vi "Configure Source Advanced Sequence Mode.vi"(0 "Instrument handle IN":refnum<k15>[](array[refnum]), 1 "Measurement Configuration":T2={"Quick Power Down"=FALSE, "Pin Name"=[], "Source Mode"=[], "Start Value"=[], "Target Value"=[], "Compliance Limit"=[], "Sense Mode"=[], "Default Ramp Rate"=[], "Ramp Rate"=[], "Start Delay"=[], "Relative To"=[], "Transient Response"=[], "Data Capture"=FALSE, "Power line frequency"=1} {"Power line frequency" items=["50 Hz", "60 Hz"]; "Start Value" format="%#_6p"; "Transient Response" items=["Slow", "Normal", "Fast"]; "Sense Mode" items=["Local Sense", "Remote Sense"]; "Relative To" items=["Power sequence start", "Previous source start", "Previous source end"]; "Target Value" format="%#_6p"; "Source Mode" items=["DC Voltage", "DC Current"]; "Start Delay" format="%#_6p"; "Compliance Limit" format="%#_6p"; "Ramp Rate" format="%#_6p"}, 2 "PowerUP?":bool, 5 "Channel Number":string[](array[string]), 7 "Ramp Configurations":T1, 11 "error in (no error)":errorcluster) -> (4 "Instrument Handle OUT":refnum<k15>[](array[refnum]), 6 "Advance Seq Created?":bool[](array[boolean]), 15 "error out":errorcluster)   [LabVIEW 2024, in "devicePowerSequencerCoreLogic.lvlib"]
uses:
  devicePowerSequencerCoreLogic.lvlib
  Measurement Configuration.ctl
  controls/Source Mode.ctl
  controls/Sense Mode.ctl
  controls/Relative To.ctl
  controls/Transient Response.ctl
  controls/Power line frequency.ctl
  controls/Ramp Configurations.ctl
  <instrlib>/niDCPower/nidcpower.llb/niDCPower Sequence Attribute Type.ctl
  <vilib>/Analysis/1siggen.llb/Ramp Pattern by Samples.vi
  <instrlib>/niDCPower/nidcpower.llb/niDCPower Create Advanced Sequence Commit Step With Channels.vi
  <instrlib>/niDCPower/nidcpower.llb/niDCPower Create Advanced Sequence Step With Channels.vi
  <vilib>/Analysis/NI_AALBase.lvlib
  Device Power Sequencer.lvlib
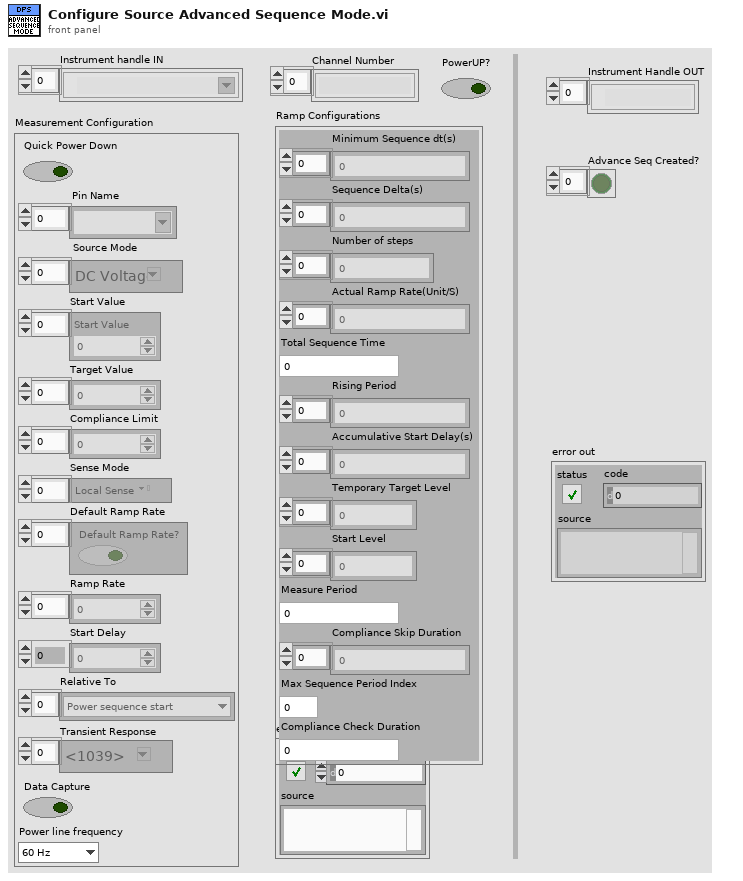
[diagram p1: front panel]
types:
  T1 = typedef "devicePowerSequencerCoreLogic.lvlib/Ramp Configurations.ctl" = cluster{"Minimum Sequence dt(s)":dbl[], "Sequence Delta(s)":dbl[], "Number of steps":i32[], "Actual Ramp Rate(Unit/S)":dbl[], "Total Sequence Time":dbl, "Rising Period":dbl[], "Accumulative Start Delay(s)":dbl[], "Temporary Target Level":dbl[], "Start Level":dbl[], "Measure Period":dbl, "Compliance Skip Duration":dbl[], "Max Sequence Period Index":i32, "Compliance Check Duration":dbl}
  T2 = typedef "Device Power Sequencer.lvlib/Measurement Configuration.ctl" = cluster{"Quick Power Down":bool, "Pin Name":string[], "Source Mode":T3[], "Start Value":dbl[], "Target Value":dbl[], "Compliance Limit":dbl[], "Sense Mode":T4[], "Default Ramp Rate":bool[], "Ramp Rate":dbl[], "Start Delay":dbl[], "Relative To":T5[], "Transient Response":T6[], "Data Capture":bool, "Power line frequency":T7}
  T3 = typedef "Device Power Sequencer.lvlib/Source Mode.ctl" = i32
  T4 = typedef "Device Power Sequencer.lvlib/Sense Mode.ctl" = i32
  T5 = typedef "Device Power Sequencer.lvlib/Relative To.ctl" = u32
  T6 = typedef "Device Power Sequencer.lvlib/Transient Response.ctl" = i32
  T7 = typedef "Device Power Sequencer.lvlib/Power line frequency.ctl" = u32
  T8 = typedef "niDCPower Sequence Attribute Type.ctl" = i32
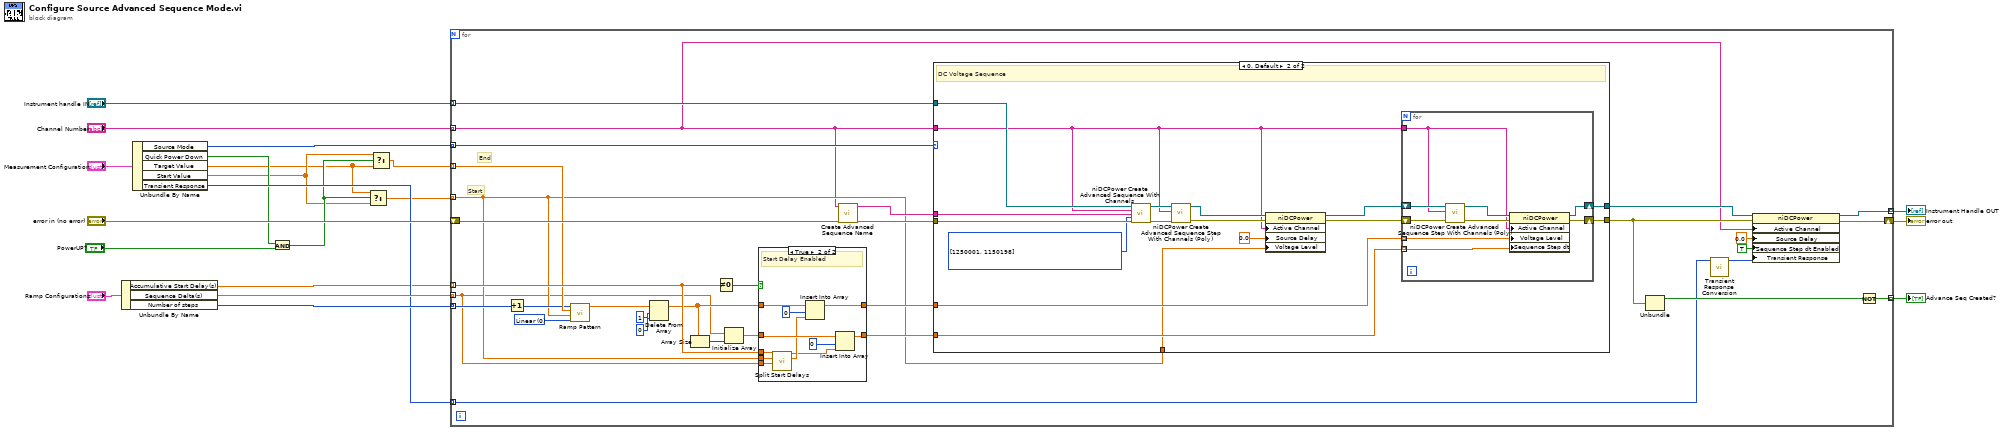
[diagram p0: block diagram]
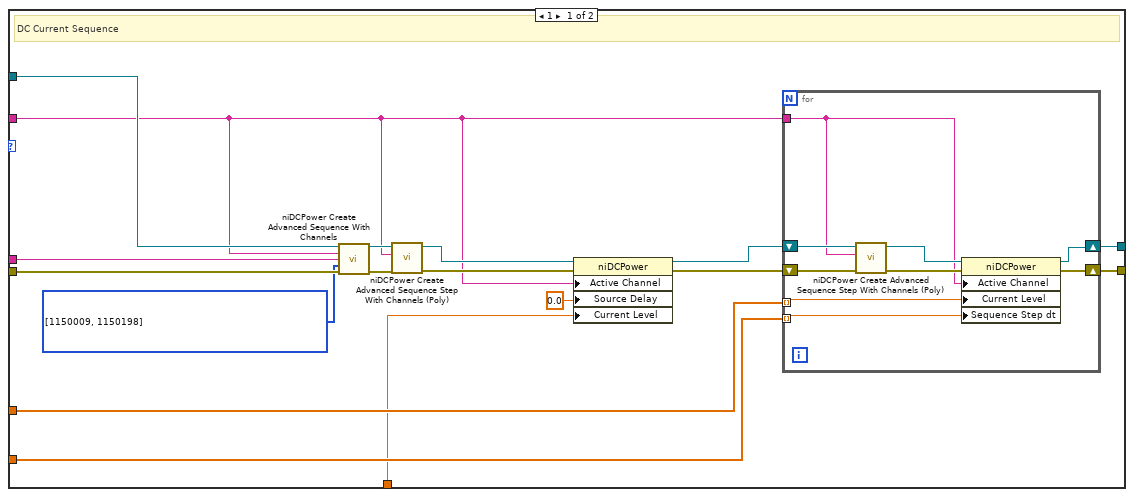
[diagram p3: hidden frame]
diagram:
  n1 = Unbundle By Name("Ramp Configurations") -> ("Accumulative Start Delay(s)"=w8:dbl[], "Sequence Delta(s)"=w15:dbl[], "Number of steps"=w17:i32[])
  n2 = Unbundle By Name("Measurement Configuration") -> ("Source Mode"=w16:T3[], "Quick Power Down"=w4:bool, "Target Value"=w1:dbl[], "Start Value"=w2:dbl[], "Transient Response"=w9:T6[])
  n3 = And(x=w4, y="PowerUP?") -> (x .and. y?=w5:bool)
  n4 = Select(t=w1, s=w5, f=w2) -> (s? t:f=w6:dbl[])
  n5 = Select(t=w2, s=w5, f=w1) -> (s? t:f=w7:dbl[])
  n6 = for {
    tunnel: "Instrument handle IN" -> [w51] mode=indexing
    tunnel: w17 -> [w52] mode=indexing
    tunnel: w7 -> [w37] mode=indexing
    tunnel: w8 -> [w38] mode=indexing
    tunnel: w16 -> [w48] mode=indexing
    tunnel: w15 -> [w22] mode=indexing
    tunnel: "Channel Number" -> [w21] mode=indexing
    shift-right: [w42] -> w12
    shift-left: "error in (no error)" -> [w44]
    tunnel: [w43] -> w11 mode=indexing
    tunnel: [w41] -> w10 mode=indexing
    tunnel: w9 -> [w27] mode=indexing
    tunnel: w6 -> [w23] mode=indexing
    w34 = u16 0 items=["Linear", "Logarithmic"] ("type")
    # "End"
    # "Start"
    n7 = Increment(x=w52) -> (x+1=w35:i32)
    n8 = call-poly <vilib>:"Ramp Pattern.vi"("type"=w34, "start"=w23, "end"=w37, "samples"=w35) -> ("Ramp Pattern"=w28:dbl[])  [unwired: 6 in, 1 out]
    n9 = Delete From Array(array=w28, length=1, index=0) -> (array with subset deleted=w31:dbl[])  [unwired: 1 out]
    n10 = Array Size(array=w31) -> (size(s)=w30:i32)
    n11 = Not Equal To 0?(x=w38) -> (x != 0?=w36:bool)
    n12 = Initialize Array(w22, w30) -> (w29:dbl[])
    n13 = case shown="True" w36 {
      tunnel: w31 -> [w54 w64]
      tunnel: [w54 w63] -> w25
      tunnel: w29 -> [w53 w60]
      tunnel: [w53 w61] -> w24
      tunnel: w38 -> [_ w59]
      tunnel: w23 -> [_ w58]
      tunnel: w22 -> [_ w55]
      frame False {
      }
      frame True {
        # "Start Delay Enabled"
        n14 = call "Split Start Delays.vi"("Start Delay"=w59, "Value"=w58, "Sequence Delta (s)"=w55) -> ("Start Delay"=w56:dbl[], "Value"=w57:dbl[])  [unwired: 11 in]
        n15 = Insert Into Array(array=w64, index=0, new element=w57) -> (w63:dbl[])
        n16 = Insert Into Array(array=w60, index=0, new element=w56) -> (w61:dbl[])
      }
    }
    n17 = call "Create Advanced Sequence Name.vi"("Channel Name"=w21, "error in (no error)"=w44) -> ("String"=w49:string, "error out"=w50:errorcluster)  [unwired: 12 in]
    n18 = case shown="0, Default" w48 {
      tunnel: w51 -> [w82 w108]
      tunnel: w50 -> [w81 w107]
      tunnel: w49 -> [w80 w106]
      tunnel: [w74 w97] -> w47
      tunnel: w25 -> [w73 w96]
      tunnel: w24 -> [w72 w95]
      tunnel: w21 -> [w66 w92]
      tunnel: [w71 w94] -> w39
      tunnel: w23 -> [w67 w93]
      frame 1 {
        w77 = T8[] [1150009, 1150198] items=["Source -> Output Function"=1150008, "Source -> Output Enabled"=1250006, "Source -> Output Resistance"=1150061, "Source -> Transient Response"=1150062, "Source -> Custom Transient Response -> Voltage Gain Bandwidth"=1150067, "Source -> Custom Transient Response -> Voltage Compensation Frequency"=1150068, "Source -> Custom Transient Response -> Voltage Pole-Zero Ratio"=1150069, "Source -> Custom Transient Response -> Current Gain Bandwidth"=1150070, "Source -> Custom Transient Response -> Current Compensation Frequency"=1150071, "Source -> Custom Transient Response -> Current Pole-Zero Ratio"=1150072, "Source -> DC Voltage -> Voltage Level"=1250001, "Source -> DC Voltage -> Voltage Level Range"=1150005, "Source -> DC Voltage -> Current Limit"=1250005, "Source -> DC Voltage -> Current Limit High"=1150187, "Source -> DC Voltage -> Current Limit Low"=1150188, "Source -> DC Voltage -> Current Limit Range"=1150004, "Source -> DC Current -> Current Level"=1150009, "Source -> DC Current -> Current Level Range"=1150011, "Source -> DC Current -> Voltage Limit"=1150010, "Source -> DC Current -> Voltage Limit High"=1150185, "Source -> DC Current -> Voltage Limit Low"=1150186, "Source -> DC Current -> Voltage Limit Range"=1150012, "Source -> Pulse Voltage -> Pulse Voltage Level"=1150080, "Source -> Pulse Voltage -> Pulse Bias Voltage Level"=1150082, "Source -> Pulse Voltage -> Pulse Voltage Level Range"=1150084, "Source -> Pulse Voltage -> Pulse Current Limit"=1150081, "Source -> Pulse Voltage -> Pulse Current Limit High"=1150193, "Source -> Pulse Voltage -> Pulse Current Limit Low"=1150194, "Source -> Pulse Voltage -> Pulse Bias Current Limit"=1150083, "Source -> Pulse Voltage -> Pulse Bias Current Limit High"=1150195, "Source -> Pulse Voltage -> Pulse Bias Current Limit Low"=1150196, "Source -> Pulse Voltage -> Pulse Current Limit Range"=1150085, "Source -> Pulse Current -> Pulse Current Level"=1150086, "Source -> Pulse Current -> Pulse Bias Current Level"=1150088, "Source -> Pulse Current -> Pulse Current Level Range"=1150090, "Source -> Pulse Current -> Pulse Voltage Limit"=1150087, "Source -> Pulse Current -> Pulse Voltage Limit High"=1150189, "Source -> Pulse Current -> Pulse Voltage Limit Low"=1150190, "Source -> Pulse Current -> Pulse Bias Voltage Limit"=1150089, "Source -> Pulse Current -> Pulse Bias Voltage Limit High"=1150191, "Source -> Pulse Current -> Pulse Bias Voltage Limit Low"=1150192, "Source -> Pulse Current -> Pulse Voltage Limit Range"=1150091, "Source -> Advanced -> Source Delay"=1150051, "Source -> Advanced -> Pulse Bias Delay"=1150092, "Source -> Advanced -> Pulse On Time"=1150093, "Source -> Advanced -> Pulse Off Time"=1150094, "Source -> Advanced -> OVP Enabled"=1250002, "Source -> Advanced -> OVP Limit"=1250003, "Source -> Advanced -> Compliance Limit Symmetry"=1150184, "Source -> Advanced -> Sequence Step Delta Time"=1150198, "Measurement -> Sense"=1150013, "Measurement -> Aperture Time"=1150058, "Measurement -> Measure Record Length"=1150063, "Measurement -> Advanced -> DC Noise Rejection"=1150066, "Measurement -> Autorange"=1150244, "Measurement -> Advanced -> Autorange Behavior"=1150245, "Measurement -> Advanced -> Autorange Aperture Time Mode"=1150246, "Measurement -> Advanced -> Autorange Minimum Aperture Time"=1150247, "Measurement -> Advanced -> Autorange Minimum Aperture Time Units"=1150248, "Measurement -> Advanced -> Autorange Minimum Current Range"=1150255, "Measurement -> Advanced -> Autorange Minimum Voltage Range"=1150256, "Measurement -> Advanced -> Autorange Threshold Mode"=1150257, "Measurement -> Advanced -> Autorange Maximum Delay After Range Change"=1150322, "LCR -> Instrument Mode"=1150208, "LCR -> Source Delay Mode"=1150315, "LCR -> Measurement Time"=1150218, "LCR -> Custom Measurement Time"=1150258, "LCR -> AC Stimulus -> Function"=1150209, "LCR -> AC Stimulus -> Frequency"=1150210, "LCR -> AC Stimulus -> Voltage Amplitude"=1150211, "LCR -> AC Stimulus -> Current Amplitude"=1150212, "LCR -> AC Stimulus -> Advanced -> Voltage Range"=1150265, "LCR -> AC Stimulus -> Advanced -> Current Range"=1150267, "LCR -> DC Bias -> Source"=1150213, "LCR -> DC Bias -> Voltage Level"=1150214, "LCR -> DC Bias -> Current Level"=1150215, "LCR -> DC Bias -> Advanced -> Voltage Range"=1150266, "LCR -> DC Bias -> Advanced -> Current Range"=1150274, "LCR -> Compensation -> Open -> Enabled"=1150220, "LCR -> Compensation -> Open -> Conductance"=1150261, "LCR -> Compensation -> Open -> Susceptance"=1150262, "LCR -> Compensation -> Short -> Enabled"=1150221, "LCR -> Compensation -> Short -> Resistance"=1150263, "LCR -> Compensation -> Short -> Reactance"=1150264, "LCR -> Compensation -> Load -> Enabled"=1150222, "LCR -> Compensation -> Load -> Measured Resistance"=1150268, "LCR -> Compensation -> Load -> Measured Reactance"=1150269, "LCR -> Compensation -> Load -> Actual Resistance"=1150270, "LCR -> Compensation -> Load -> Actual Reactance"=1150271, "LCR -> Impedance Range -> Impedance Range"=1150217, "LCR -> Impedance Range -> Impedance Autorange"=1150216, "LCR -> Impedance Range -> Advanced -> Impedance Range Source"=1150321, "LCR -> Impedance Range -> Advanced -> Load Resistance"=1150318, "LCR -> Impedance Range -> Advanced -> Load Inductance"=1150319, "LCR -> Impedance Range -> Advanced -> Load Capacitance"=1150320] ("advanced sequence properties")
        # "DC Current Sequence"
        n19 = call <instrlib>:"niDCPower Create Advanced Sequence With Channels.vi"("instrument handle"=w82, "channel name"=w66, "sequence name"=w80, "advanced sequence properties"=w77, "error in (no error)"=w81) -> ("instrument handle out"=w78:refnum<k15>, "error out"=w79:errorcluster)  [unwired: 9 in]
        n20 = call-poly <instrlib>:"niDCPower Create Advanced Sequence Step With Channels (Poly).vi"("error in (no error)"=w79, "channel name"=w66, "instrument handle"=w78) -> ("error out"=w69:errorcluster, "instrument handle out"=w70:refnum<k15>)  [unwired: 7 in]
        n21 = property class="niDCPower"(reference=w70, error in=w69, "Active Channel"=w66, "Source Delay"=0.0 ("Source:Advanced:Source Delay"), "Current Level"=w67) -> (reference out=w75:refnum<k15>, error out=w76:errorcluster)
        n22 = for {
          shift-right: [w87] -> w71
          shift-left: w76 -> [w90]
          shift-right: [w86] -> w74
          shift-left: w75 -> [w91]
          tunnel: w73 -> [w85] mode=indexing
          tunnel: w72 -> [w84] mode=indexing
          tunnel: w66 -> [w83]
          n23 = call-poly <instrlib>:"niDCPower Create Advanced Sequence Step With Channels (Poly).vi"("error in (no error)"=w90, "channel name"=w83, "instrument handle"=w91) -> ("error out"=w88:errorcluster, "instrument handle out"=w89:refnum<k15>)  [unwired: 7 in]
          n24 = property class="niDCPower"(reference=w89, error in=w88, "Active Channel"=w83, "Current Level"=w85, "Sequence Step dt"=w84) -> (reference out=w86:refnum<k15>, error out=w87:errorcluster)
        }
      }
      frame 0, Default {
        w103 = T8[] [1250001, 1150198] items=["Source -> Output Function"=1150008, "Source -> Output Enabled"=1250006, "Source -> Output Resistance"=1150061, "Source -> Transient Response"=1150062, "Source -> Custom Transient Response -> Voltage Gain Bandwidth"=1150067, "Source -> Custom Transient Response -> Voltage Compensation Frequency"=1150068, "Source -> Custom Transient Response -> Voltage Pole-Zero Ratio"=1150069, "Source -> Custom Transient Response -> Current Gain Bandwidth"=1150070, "Source -> Custom Transient Response -> Current Compensation Frequency"=1150071, "Source -> Custom Transient Response -> Current Pole-Zero Ratio"=1150072, "Source -> DC Voltage -> Voltage Level"=1250001, "Source -> DC Voltage -> Voltage Level Range"=1150005, "Source -> DC Voltage -> Current Limit"=1250005, "Source -> DC Voltage -> Current Limit High"=1150187, "Source -> DC Voltage -> Current Limit Low"=1150188, "Source -> DC Voltage -> Current Limit Range"=1150004, "Source -> DC Current -> Current Level"=1150009, "Source -> DC Current -> Current Level Range"=1150011, "Source -> DC Current -> Voltage Limit"=1150010, "Source -> DC Current -> Voltage Limit High"=1150185, "Source -> DC Current -> Voltage Limit Low"=1150186, "Source -> DC Current -> Voltage Limit Range"=1150012, "Source -> Pulse Voltage -> Pulse Voltage Level"=1150080, "Source -> Pulse Voltage -> Pulse Bias Voltage Level"=1150082, "Source -> Pulse Voltage -> Pulse Voltage Level Range"=1150084, "Source -> Pulse Voltage -> Pulse Current Limit"=1150081, "Source -> Pulse Voltage -> Pulse Current Limit High"=1150193, "Source -> Pulse Voltage -> Pulse Current Limit Low"=1150194, "Source -> Pulse Voltage -> Pulse Bias Current Limit"=1150083, "Source -> Pulse Voltage -> Pulse Bias Current Limit High"=1150195, "Source -> Pulse Voltage -> Pulse Bias Current Limit Low"=1150196, "Source -> Pulse Voltage -> Pulse Current Limit Range"=1150085, "Source -> Pulse Current -> Pulse Current Level"=1150086, "Source -> Pulse Current -> Pulse Bias Current Level"=1150088, "Source -> Pulse Current -> Pulse Current Level Range"=1150090, "Source -> Pulse Current -> Pulse Voltage Limit"=1150087, "Source -> Pulse Current -> Pulse Voltage Limit High"=1150189, "Source -> Pulse Current -> Pulse Voltage Limit Low"=1150190, "Source -> Pulse Current -> Pulse Bias Voltage Limit"=1150089, "Source -> Pulse Current -> Pulse Bias Voltage Limit High"=1150191, "Source -> Pulse Current -> Pulse Bias Voltage Limit Low"=1150192, "Source -> Pulse Current -> Pulse Voltage Limit Range"=1150091, "Source -> Advanced -> Source Delay"=1150051, "Source -> Advanced -> Pulse Bias Delay"=1150092, "Source -> Advanced -> Pulse On Time"=1150093, "Source -> Advanced -> Pulse Off Time"=1150094, "Source -> Advanced -> OVP Enabled"=1250002, "Source -> Advanced -> OVP Limit"=1250003, "Source -> Advanced -> Compliance Limit Symmetry"=1150184, "Source -> Advanced -> Sequence Step Delta Time"=1150198, "Measurement -> Sense"=1150013, "Measurement -> Aperture Time"=1150058, "Measurement -> Measure Record Length"=1150063, "Measurement -> Advanced -> DC Noise Rejection"=1150066, "Measurement -> Autorange"=1150244, "Measurement -> Advanced -> Autorange Behavior"=1150245, "Measurement -> Advanced -> Autorange Aperture Time Mode"=1150246, "Measurement -> Advanced -> Autorange Minimum Aperture Time"=1150247, "Measurement -> Advanced -> Autorange Minimum Aperture Time Units"=1150248, "Measurement -> Advanced -> Autorange Minimum Current Range"=1150255, "Measurement -> Advanced -> Autorange Minimum Voltage Range"=1150256, "Measurement -> Advanced -> Autorange Threshold Mode"=1150257, "Measurement -> Advanced -> Autorange Maximum Delay After Range Change"=1150322, "LCR -> Instrument Mode"=1150208, "LCR -> Source Delay Mode"=1150315, "LCR -> Measurement Time"=1150218, "LCR -> Custom Measurement Time"=1150258, "LCR -> AC Stimulus -> Function"=1150209, "LCR -> AC Stimulus -> Frequency"=1150210, "LCR -> AC Stimulus -> Voltage Amplitude"=1150211, "LCR -> AC Stimulus -> Current Amplitude"=1150212, "LCR -> AC Stimulus -> Advanced -> Voltage Range"=1150265, "LCR -> AC Stimulus -> Advanced -> Current Range"=1150267, "LCR -> DC Bias -> Source"=1150213, "LCR -> DC Bias -> Voltage Level"=1150214, "LCR -> DC Bias -> Current Level"=1150215, "LCR -> DC Bias -> Advanced -> Voltage Range"=1150266, "LCR -> DC Bias -> Advanced -> Current Range"=1150274, "LCR -> Compensation -> Open -> Enabled"=1150220, "LCR -> Compensation -> Open -> Conductance"=1150261, "LCR -> Compensation -> Open -> Susceptance"=1150262, "LCR -> Compensation -> Short -> Enabled"=1150221, "LCR -> Compensation -> Short -> Resistance"=1150263, "LCR -> Compensation -> Short -> Reactance"=1150264, "LCR -> Compensation -> Load -> Enabled"=1150222, "LCR -> Compensation -> Load -> Measured Resistance"=1150268, "LCR -> Compensation -> Load -> Measured Reactance"=1150269, "LCR -> Compensation -> Load -> Actual Resistance"=1150270, "LCR -> Compensation -> Load -> Actual Reactance"=1150271, "LCR -> Impedance Range -> Impedance Range"=1150217, "LCR -> Impedance Range -> Impedance Autorange"=1150216, "LCR -> Impedance Range -> Advanced -> Impedance Range Source"=1150321, "LCR -> Impedance Range -> Advanced -> Load Resistance"=1150318, "LCR -> Impedance Range -> Advanced -> Load Inductance"=1150319, "LCR -> Impedance Range -> Advanced -> Load Capacitance"=1150320] ("advanced sequence properties")
        # "DC Voltage Sequence"
        n25 = call <instrlib>:"niDCPower Create Advanced Sequence With Channels.vi"("instrument handle"=w108, "channel name"=w92, "sequence name"=w106, "advanced sequence properties"=w103, "error in (no error)"=w107) -> ("instrument handle out"=w104:refnum<k15>, "error out"=w105:errorcluster)  [unwired: 9 in]
        n26 = call-poly <instrlib>:"niDCPower Create Advanced Sequence Step With Channels (Poly).vi"("error in (no error)"=w105, "channel name"=w92, "instrument handle"=w104) -> ("error out"=w101:errorcluster, "instrument handle out"=w102:refnum<k15>)  [unwired: 7 in]
        n27 = property class="niDCPower"(reference=w102, error in=w101, "Active Channel"=w92, "Source Delay"=0.0 ("Source:Advanced:Source Delay"), "Voltage Level"=w93) -> (reference out=w98:refnum<k15>, error out=w99:errorcluster)
        n28 = for {
          shift-right: [w113] -> w94
          shift-left: w99 -> [w116]
          shift-right: [w112] -> w97
          shift-left: w98 -> [w117]
          tunnel: w96 -> [w111] mode=indexing
          tunnel: w95 -> [w110] mode=indexing
          tunnel: w92 -> [w109]
          n29 = call-poly <instrlib>:"niDCPower Create Advanced Sequence Step With Channels (Poly).vi"("error in (no error)"=w116, "channel name"=w109, "instrument handle"=w117) -> ("error out"=w114:errorcluster, "instrument handle out"=w115:refnum<k15>)  [unwired: 7 in]
          n30 = property class="niDCPower"(reference=w115, error in=w114, "Active Channel"=w109, "Voltage Level"=w111, "Sequence Step dt"=w110) -> (reference out=w112:refnum<k15>, error out=w113:errorcluster)
        }
      }
    }
    n31 = Unbundle(w39) -> ("status"=w40:bool)  [unwired: 2 out]
    n32 = call "Transient Response Conversion.vi"("Trans Resp"=w27) -> ("Source:Transient Response"=w26:i32)  [unwired: 14 in]
    n33 = property class="niDCPower"(reference=w47, error in=w39, "Active Channel"=w21, "Source Delay"=0.0 ("Source:Advanced:Source Delay"), "Sequence Step dt Enabled"=TRUE ("Source:Advanced:Sequence Step Delta Time Enabled"), "Transient Response"=w26) -> (reference out=w43:refnum<k15>, error out=w42:errorcluster)
    n34 = Not(x=w40) -> (.not. x?=w41:bool)
  }
  "error out" <- w12
  "Instrument Handle OUT" <- w11
  "Advance Seq Created?" <- w10
